vi "Bass Subvi2.vi"(0 "Image Dst Out":T2) -> (9 "Orange Bass LED":bool, 11 "Red Bass LED":bool, 13 "Green Bass LED":bool, 15 "Yellow Bass LED":bool, 19 "Blue Bass LED":bool)   [LabVIEW 2009]
uses:
  <vilib>/vision/Image Controls.llb/IMAQ Image.ctl
  <vilib>/Analysis/3filter.llb/Filter Passband Type.ctl
  <vilib>/Analysis/3filter.llb/Butterworth Filter (DBL).vi
  <vilib>/Analysis/NI_AALBase.lvlib
  <vilib>/vision/NI_Vision_Development_Module.lvlib
panel:
  in  "Blue Bass 2":T1={"Global Rectangle"=[192, 292, 199, 386], "Contours"=[{"ID"=enum."External", "Type"=2, "Coordinates"=[192, 385, 198, 292]}]} {"Contours"."Type" items=["No Selection", "Point", "Line", "Rectangle", "Oval", "Polygon", "Freehand Region", "Annulus", "Unused2", "Unused3", "Broken Line", "Freehand Line", "Rotated Rectangle"]}
  in  "Orange Bass 2":T1={"Global Rectangle"=[220, 302, 227, 392], "Contours"=[{"ID"=enum."External", "Type"=2, "Coordinates"=[226, 391, 220, 302]}]} {"Contours"."Type" items=["No Selection", "Point", "Line", "Rectangle", "Oval", "Polygon", "Freehand Region", "Annulus", "Unused2", "Unused3", "Broken Line", "Freehand Line", "Rotated Rectangle"]}
  in  "Green Bass 2":T1={"Global Rectangle"=[100, 292, 131, 371], "Contours"=[{"ID"=enum."External", "Type"=2, "Coordinates"=[100, 370, 130, 292]}]} {"Contours"."Type" items=["No Selection", "Point", "Line", "Rectangle", "Oval", "Polygon", "Freehand Region", "Annulus", "Unused2", "Unused3", "Broken Line", "Freehand Line", "Rotated Rectangle"]}
  in  "Red Bass 2":T1={"Global Rectangle"=[129, 294, 154, 376], "Contours"=[{"ID"=enum."External", "Type"=2, "Coordinates"=[129, 375, 153, 294]}]} {"Contours"."Type" items=["No Selection", "Point", "Line", "Rectangle", "Oval", "Polygon", "Freehand Region", "Annulus", "Unused2", "Unused3", "Broken Line", "Freehand Line", "Rotated Rectangle"]}
  in  "Yellow Bass 2":T1={"Global Rectangle"=[160, 295, 175, 378], "Contours"=[{"ID"=enum."External", "Type"=2, "Coordinates"=[160, 377, 174, 295]}]} {"Contours"."Type" items=["No Selection", "Point", "Line", "Rectangle", "Oval", "Polygon", "Freehand Region", "Annulus", "Unused2", "Unused3", "Broken Line", "Freehand Line", "Rotated Rectangle"]}
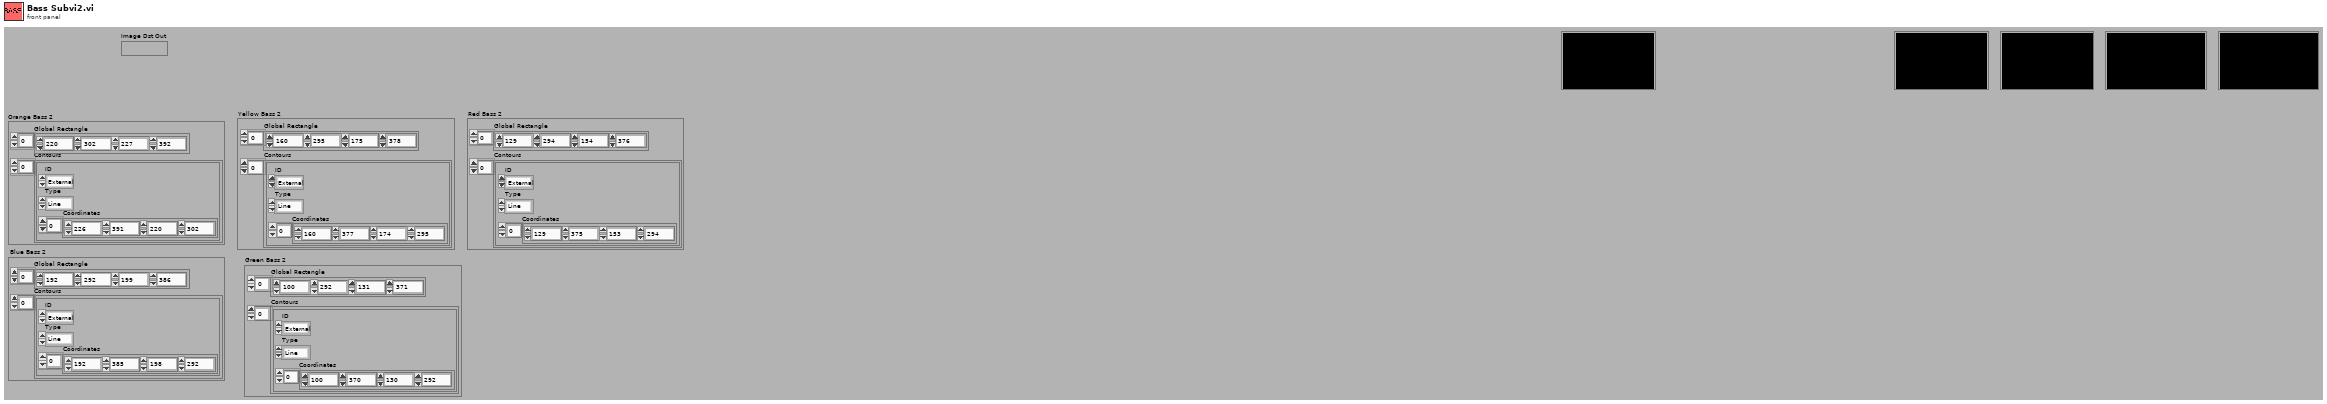
[diagram p1: front panel]
types:
  T1 = cluster{"Global Rectangle":i32[], "Contours":cluster{"ID":enum32{"External", "Internal"}, "Type":u32, "Coordinates":i32[]}[]}
  T2 = typedef "IMAQ Image.ctl" = refnum<image>
  T3 = typedef "NI_AALBase.lvlib/Filter Passband Type.ctl" = enum32{"Lowpass", "Highpass", "Bandpass", "Bandstop"}
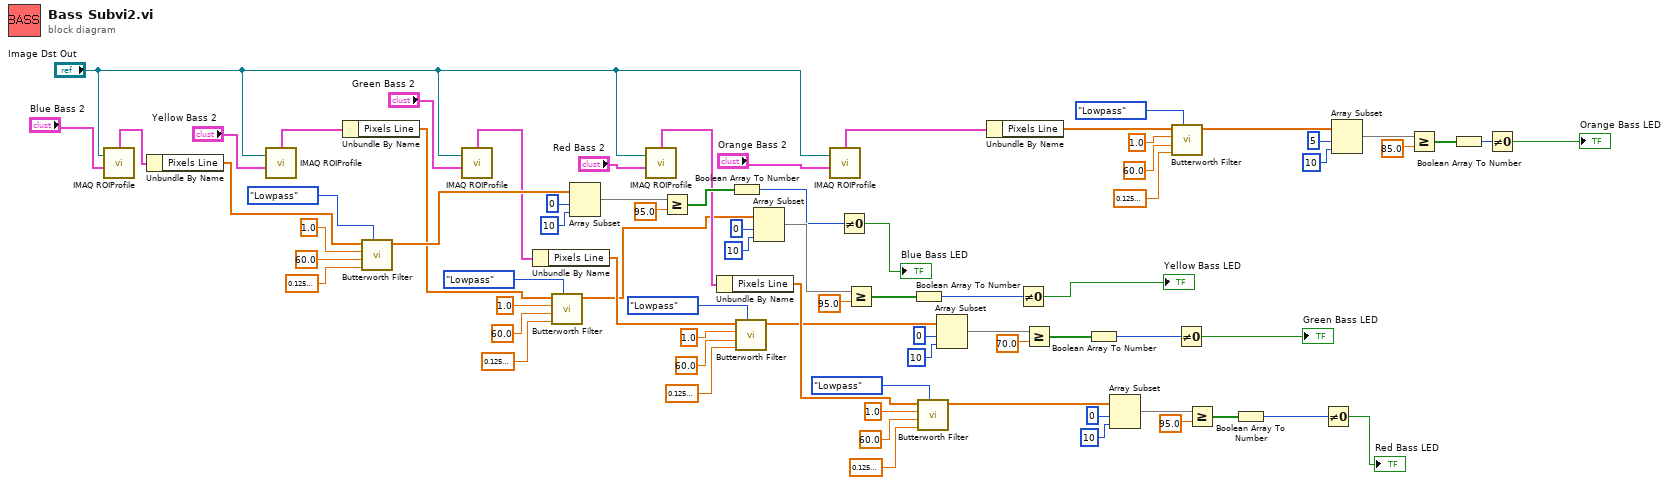
[diagram p0: block diagram]
diagram:
  n1 = call "IMAQ ROIProfile"("ROI Descriptor"="Blue Bass 2", "Image"="Image Dst Out") -> ("ROI Graph"=w26:cluster{"x0":sgl, "dx":sgl, "Pixels Line":sgl[]})  [unwired: 1 in, 5 out]
  n2 = Unbundle By Name(w26) -> ("Pixels Line"=w4:sgl[])
  n3 = call "IMAQ ROIProfile"("ROI Descriptor"="Yellow Bass 2", "Image"="Image Dst Out") -> ("ROI Graph"=w23:cluster{"x0":sgl, "dx":sgl, "Pixels Line":sgl[]})  [unwired: 1 in, 5 out]
  n4 = Unbundle By Name(w23) -> ("Pixels Line"=w20:sgl[])
  n5 = call-poly <vilib>:"Butterworth Filter.vi"("filter type"=Filter_Passband_Type."Lowpass", "low cutoff freq: fl"=0.12500000000000006 ("low 2"), "high cutoff freq: fh"=60.0 ("high 8"), "sampling freq: fs"=1.0 ("sampling  8"), "X"=w4) -> ("Filtered X"=w40:dbl[])  [unwired: 3 in, 1 out]
  n6 = call "IMAQ ROIProfile"("ROI Descriptor"="Green Bass 2", "Image"="Image Dst Out") -> ("ROI Graph"=w28:cluster{"x0":sgl, "dx":sgl, "Pixels Line":sgl[]})  [unwired: 1 in, 5 out]
  n7 = Unbundle By Name(w28) -> ("Pixels Line"=w31:sgl[])
  n8 = call-poly <vilib>:"Butterworth Filter.vi"("filter type"=Filter_Passband_Type."Lowpass", "low cutoff freq: fl"=0.12500000000000006 ("low  7"), "high cutoff freq: fh"=60.0 ("high 7"), "sampling freq: fs"=1.0 ("sampling 7"), "X"=w20) -> ("Filtered X"=w24:dbl[])  [unwired: 3 in, 1 out]
  n9 = Array Subset(array=w40, index=0, length=10) -> (w10:dbl[])
  n10 = call "IMAQ ROIProfile"("ROI Descriptor"="Red Bass 2", "Image"="Image Dst Out") -> ("ROI Graph"=w52:cluster{"x0":sgl, "dx":sgl, "Pixels Line":sgl[]})  [unwired: 1 in, 5 out]
  n11 = Greater Or Equal?(x=w10, y=95.0) -> (x >= y?=w75:bool[])
  n12 = Unbundle By Name(w52) -> ("Pixels Line"=w49:sgl[])
  n13 = Boolean Array To Number(Boolean array=w75) -> (number=w12:u32)
  n14 = call-poly <vilib>:"Butterworth Filter.vi"("filter type"=Filter_Passband_Type."Lowpass", "low cutoff freq: fl"=0.12500000000000006 ("low  6"), "high cutoff freq: fh"=60.0 ("high 6"), "sampling freq: fs"=1.0 ("sampling 6"), "X"=w31) -> ("Filtered X"=w27:dbl[])  [unwired: 3 in, 1 out]
  n15 = Array Subset(array=w24, index=0, length=10) -> (w15:dbl[])
  n16 = call "IMAQ ROIProfile"("ROI Descriptor"="Orange Bass 2", "Image"="Image Dst Out") -> ("ROI Graph"=w58:cluster{"x0":sgl, "dx":sgl, "Pixels Line":sgl[]})  [unwired: 1 in, 5 out]
  n17 = Not Equal To 0?(x=w12) -> (x != 0?=→"Blue Bass LED":bool)
  n18 = Greater Or Equal?(x=w15, y=95.0) -> (x >= y?=w17:bool[])
  n19 = Boolean Array To Number(Boolean array=w17) -> (number=w18:u32)
  n20 = call-poly <vilib>:"Butterworth Filter.vi"("filter type"=Filter_Passband_Type."Lowpass", "low cutoff freq: fl"=0.12500000000000006 ("low  5"), "high cutoff freq: fh"=60.0 ("high 5"), "sampling freq: fs"=1.0 ("sampling 5"), "X"=w49) -> ("Filtered X"=w53:dbl[])  [unwired: 3 in, 1 out]
  n21 = Array Subset(array=w27, index=0, length=10) -> (w36:dbl[])
  n22 = Unbundle By Name(w58) -> ("Pixels Line"=w61:sgl[])
  n23 = Not Equal To 0?(x=w18) -> (x != 0?=→"Yellow Bass LED":bool)
  n24 = Greater Or Equal?(x=w36, y=70.0) -> (x >= y?=w34:bool[])
  n25 = Boolean Array To Number(Boolean array=w34) -> (number=w33:u32)
  n26 = Array Subset(array=w53, index=0, length=10) -> (w44:dbl[])
  n27 = call-poly <vilib>:"Butterworth Filter.vi"("filter type"=Filter_Passband_Type."Lowpass", "low cutoff freq: fl"=0.12500000000000006 ("low  8"), "high cutoff freq: fh"=60.0 ("high 9"), "sampling freq: fs"=1.0 ("sampling 8"), "X"=w61) -> ("Filtered X"=w57:dbl[])  [unwired: 3 in, 1 out]
  n28 = Not Equal To 0?(x=w33) -> (x != 0?=→"Green Bass LED":bool)
  n29 = Greater Or Equal?(x=w44, y=95.0) -> (x >= y?=w46:bool[])
  n30 = Boolean Array To Number(Boolean array=w46) -> (number=w47:u32)
  n31 = Not Equal To 0?(x=w47) -> (x != 0?=→"Red Bass LED":bool)
  n32 = Array Subset(array=w57, index=5, length=10) -> (w66:dbl[])
  n33 = Greater Or Equal?(x=w66, y=85.0) -> (x >= y?=w64:bool[])
  n34 = Boolean Array To Number(Boolean array=w64) -> (number=w63:u32)
  n35 = Not Equal To 0?(x=w63) -> (x != 0?=→"Orange Bass LED":bool)
